vi "GetAngleSetpoint.vi"(8 "error in (no error)":errorcluster) -> (0 "error out":errorcluster, 2 "angleSepointOutput":dbl)   [LabVIEW 2016, in "DriveBase.lvclass"]
uses:
  DriveBase.lvclass
  DriveBase.lvclass/DriveBase.ctl
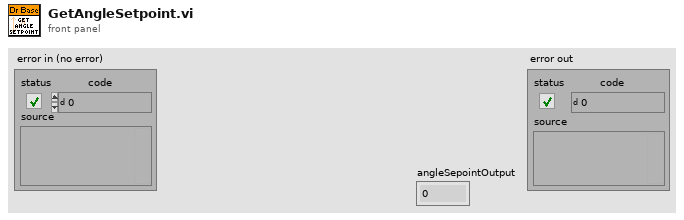
[diagram p1: front panel]
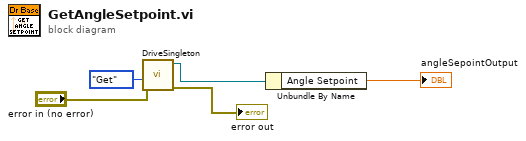
[diagram p0: block diagram]
diagram:
  n1 = call "DriveSingleton.vi"("error in (no error)"="error in (no error)", "Get/Set"=enum16{"Get", "Set"}."Get") -> ("error out"=→"error out":errorcluster, "DriveBase.lvclass 2"=w4:refnum<class "DriveBase.lvclass">)  [unwired: 8 in]
  n2 = Unbundle By Name(w4) -> ("Angle Setpoint"=→"angleSepointOutput":dbl)
